vi "Control_Tiempo_UV_Lamp.vi"(0 "Refnum in":refnum<k21>, 1 "Toff":u32=10 caption="Tiempo OFF (UV_Lamp)" min=10 max=120 step=1, 2 "TOn":u32=10 caption="Tiempo ON (UV_Lamp)" min=1 max=60 step=1, 5 "error in":errorcluster) -> (19 "error out":errorcluster)   [LabVIEW 2013]
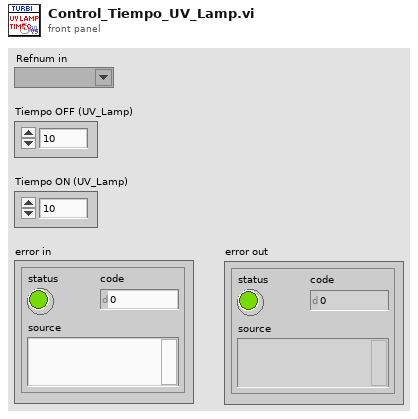
[diagram p1: front panel]
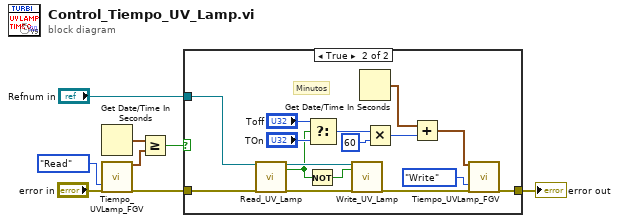
[diagram p0: block diagram]
diagram:
  n1 = Get Date/Time In Seconds() -> (seconds since 1Jan1904=w2:timestamp)
  n2 = call "Tiempo_UVLamp_FGV.vi"("Opción"=enum16{"Write", "Read"}."Read", "Error In"="error in") -> ("Tiempo_OUT"=w1:timestamp, "Error Out"=w6:errorcluster)  [unwired: 16 in]
  n3 = Greater Or Equal?(x=w2, y=w1) -> (x >= y?=w5:bool)
  n4 = case shown="True" w5 {
    tunnel: w6 -> [w9 w25]
    tunnel: "Refnum in" -> [_ w24]
    tunnel: [w9 w10] -> w8
    frame False {
    }
    frame True {
      # "Minutos"
      n5 = call "Read_UV_Lamp.vi"("Refnum in"=w24, "error in (no error)"=w25) -> ("Refnum out"=w21:refnum<k21>, "On/Off?"=w16:bool, "error out"=w22:errorcluster)  [unwired: 15 in]
      n6 = Not(x=w16) -> (.not. x?=w23:bool)
      n7 = Select(t="Toff", s=w16, f="TOn") -> (s? t:f=w13:u32)
      n8 = call "Write_UV_Lamp.vi"("Refnum in"=w21, "On/Off"=w23, "error in (no error)"=w22) -> ("error out"=w20:errorcluster)  [unwired: 15 in, 1 out]
      n9 = Get Date/Time In Seconds() -> (seconds since 1Jan1904=w15:timestamp)
      n10 = Multiply(x=w13, y=u32 60) -> (x*y=w14:u32)
      n11 = Add(x=w15, y=w14) -> (x+y=w11:timestamp)
      n12 = call "Tiempo_UVLamp_FGV.vi"("Tiempo_IN"=w11, "Opción"=enum16{"Write", "Read"}."Write", "Error In"=w20) -> ("Error Out"=w10:errorcluster)  [unwired: 15 in, 1 out]
    }
  }
  "error out" <- w8
